vi "Write Settings XML.vi"(8 "error in (no error)":errorcluster, 9 "Tweezertron Ctrl Refs":T1, 10 "name or relative path":string, 11 "path":path) -> (0 "error out":errorcluster)   [LabVIEW 2020]
uses:
  _Controls/Tweezertron Ctrl Refs.ctl
  _Controls/Confocal Controls.ctl
  _Controls/iFlex.ctl
  _Controls/PIFOC Position.ctl
  _Controls/Manlight Controls.ctl
  _Controls/Exp Params.ctl
  _Controls/Image Thresholds.ctl
  <vilib>/Utility/xml.llb/Write to XML File(string).vi
panel:
  out "XML String":string
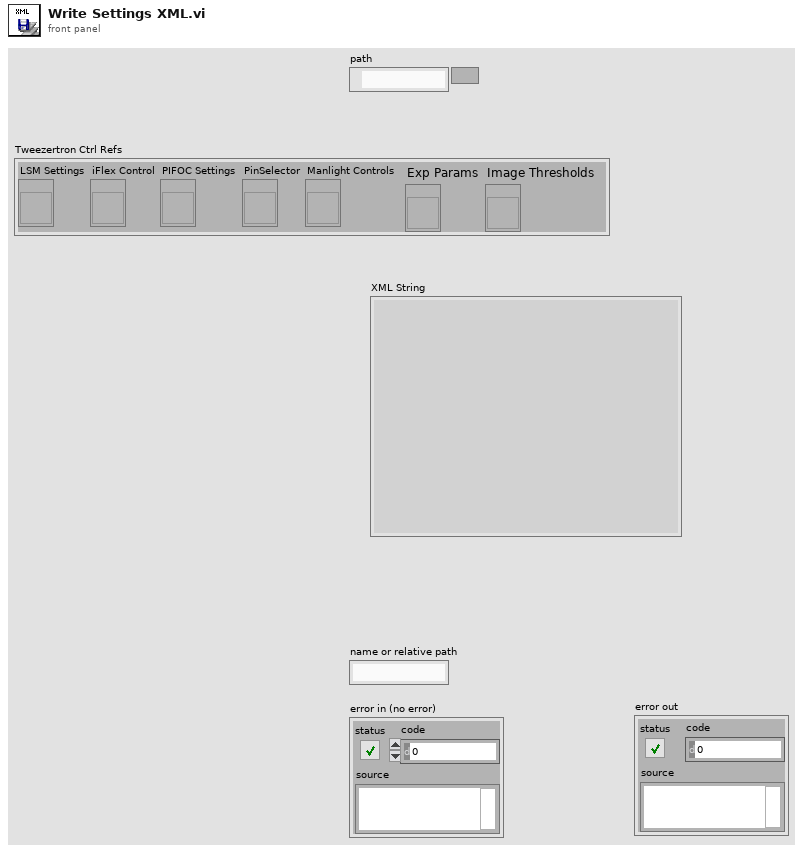
[diagram p1: front panel]
types:
  T1 = typedef "Tweezertron Ctrl Refs.ctl" = cluster{"LSM Settings":refnum<vi>, "iFlex Control":refnum<vi>, "PIFOC Settings":refnum<vi>, "PinSelector":refnum<vi>, "Manlight Controls":refnum<vi>, "Exp Params":refnum<vi>, "Image Thresholds":refnum<vi>}
  T2 = typedef "Confocal Controls.ctl" = cluster{"Channel Selection":enum32{"A", "B", "AB"}, "Pixel Count":cluster{"Pixels in X":u32, "Pixels in Y":u32}, "Field Size":dbl, "Frames":u8, "Averaging":bool, "Alignment":dbl, "Scan Mode":bool, "Gain":cluster{"Gain A":u8, "Gain B":u8}, "Enable PMTs":cluster{"A":bool, "B":bool}, "Voltage Range":cluster{"Range A":u16, "Range B":u16}, "Multi Frame Count":dbl, "Trigger Mode":dbl, "Real Time Averaging":bool, "PFOV":dbl, "MicronsPerPx":dbl}
  T3 = typedef "iFlex.ctl" = cluster{"Power 561":dbl, "Power 488":dbl, "Global Shutter":bool, "561 Shutter":bool}
  T4 = typedef "PIFOC Position.ctl" = cluster{"PIFOC Position (mm) [SET]":dbl, "PIFOC Position\n(um) [ACT]":dbl, "last command":string}
  T5 = typedef "Manlight Controls.ctl" = cluster{"Manlight Power":dbl, "Open Serial":bool, "VISA Refnum":refnum<visa-resource-name>}
  T6 = typedef "Exp Params.ctl" = cluster{"Experiment Type":string, "Experiment Name":string, "ExpPath":path, "TSFrames":i32, "TSfps":i32, "ZTSFrames":i32, "ZTSdt":i32, "Streaming":bool, "Z Stack Settings":cluster{"Start":dbl, "Step Size":dbl, "Finish":dbl}, "total images":i32, "tdms ref":refnum<k34>, "frame #":i64, "images per stack":i32, "total stacks":i32, "period":i32, "PI MVR Increment":string}
  T7 = cluster{"Value":T2, "Value":T3, "Value":T4, "Value":dbl, "Value":T5, "Value":T6}
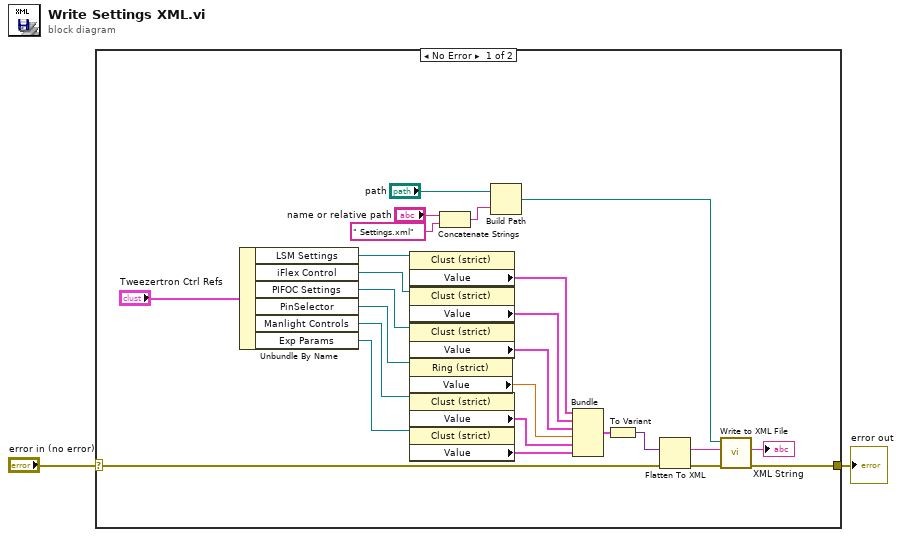
[diagram p0: block diagram]
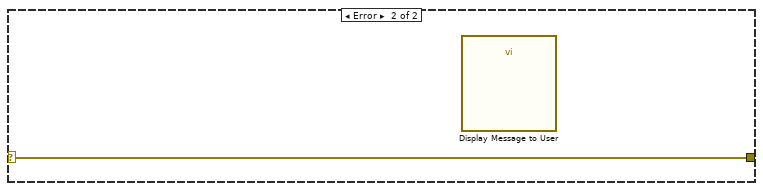
[diagram p2: hidden frame]
diagram:
  n1 = case shown="No Error" "error in (no error)" {
    selector: "error in (no error)" -> [w25 w27]
    tunnel: [w22 w27] -> w1
    frame No Error {
      n2 = Unbundle By Name("Tweezertron Ctrl Refs") -> ("LSM Settings"=w19:refnum<vi>, "iFlex Control"=w20:refnum<vi>, "PIFOC Settings"=w21:refnum<vi>, "PinSelector"=w13:refnum<vi>, "Manlight Controls"=w10:refnum<vi>, "Exp Params"=w8:refnum<vi>)
      n3 = property on="Property Node" class="Clust (strict)"(reference=w19) -> ("Value"=w16:T2)  [unwired: 1 in, 2 out]
      n4 = property on="Property Node" class="Clust (strict)"(reference=w20) -> ("Value"=w18:T3)  [unwired: 1 in, 2 out]
      n5 = property on="Property Node" class="Clust (strict)"(reference=w21) -> ("Value"=w17:T4)  [unwired: 1 in, 2 out]
      n6 = property on="Property Node" class="Ring (strict)"(reference=w13) -> ("Value"=w12:dbl)  [unwired: 1 in, 2 out]
      n7 = property on="Property Node" class="Clust (strict)"(reference=w10) -> ("Value"=w9:T5)  [unwired: 1 in, 2 out]
      n8 = property on="Property Node" class="Clust (strict)"(reference=w8) -> ("Value"=w7:T6)  [unwired: 1 in, 2 out]
      n9 = Concatenate Strings("name or relative path", " Settings.xml" ("string")) -> (w5:string)
      n10 = Build Path(base path="path", name or relative path=w5) -> (appended path=w26:path)
      n11 = Bundle("Value"=w16, "Value"=w18, "Value"=w17, "Value"=w12, "Value"=w9, "Value"=w7) -> (w15:T7)  [unwired: 1 in]
      n12 = To Variant(anything=w15) -> (Variant=w14:variant)
      n13 = Flatten To XML(6:w14) -> (2:w23:string)
      n14 = call-poly <vilib>:"Write to XML File.vi"("error in (no error)"=w25, "XML Input"=w23, "XML File Path"=w26) -> ("error out"=w22:errorcluster, "XML String"=→"XML String":string)  [unwired: 6 in, 1 out]
    }
    frame Error {
      n15 = call "Display Message to User"() -> ()  [unwired: 10 in, 2 out]
    }
  }
  "error out" <- w1
